vi "Array of VData to VArray__ogtk.vi"(7 "Array Name":string, 8 "error in (no error)":errorcluster, 9 "Element Type (when empty)":variant, 10 "1D Array of VData":variant[](array[variant])) -> (0 "error out":errorcluster, 2 "VArray":variant)   [LabVIEW 2023, in "openg_variant.lvlib"]
doc: "Converts a 1D Array of variants (of identical element datatypes) to an array of data wrapped in a Variant."
uses:
  openg_variant.lvlib
  error/error.llb/openg_error.lvlib
panel:
  # "[OpenG VI Tags] ***Do Not Remove***"
  # "Array of VData to VArray.vi\n\nConverts a 1D Array of variants (of identical element datatypes) to an array of \n\nPlease visit http://www.OpenG.org to learn about the\nOpen Source LabVIEW software movement.\n\nNOTICE -- YOU MUST LEAVE THIS NOTICE IN PLACE.  PER THE TERMS OF THE LICENSE BELOW, YOU MAY SUBLICENSE THIS SOFTWARE \nIN ANY WAY THAT DOES NOT CONFLICT WITH THIS LICENSE.\n\n### BSD License (http://www.opensource.org/licenses/bsd-license.php) Begin ###\n \nCopyright (c) 2002, Jean-Pierre Drolet <drolet_jp@hotmail.com>\nCopyright (c) 2002-2006, Jim Kring <jim@jimkring.com>\n\nAll rights reserved.\n\nRedistribution and use in source and binary forms, with or without modification, are permitted provided that the following conditions are met:\n\n    * Redistributions of source code must retain the above copyright notice, this list of conditions and the following disclaimer.\n    * Redistributions in binary form must reproduce the above copyright notice, this list of conditions and the following disclaimer in the \n       documentation and/or other materials provided with the distribution.\n    * Neither the name of SciWare, James Kring, Inc., nor the names of its contributors may be used to endorse or promote products derived \n       from this software without specific prior written permission.\n\nTHIS SOFTWARE IS PROVIDED BY THE COPYRIGHT HOLDERS AND CONTRIBUTORS \"AS IS\" AND ANY EXPRESS OR IMPLIED WARRANTIES, \nINCLUDING, BUT NOT LIMITED TO, THE IMPLIED WARRANTIES OF MERCHANTABILITY AND FITNESS FOR A PARTICULAR PURPOSE ARE \nDISCLAIMED. IN NO EVENT SHALL THE COPYRIGHT OWNER OR CONTRIBUTORS BE LIABLE FOR ANY DIRECT, INDIRECT, INCIDENTAL,\n SPECIAL, EXEMPLARY, OR CONSEQUENTIAL DAMAGES (INCLUDING, BUT NOT LIMITED TO, PROCUREMENT OF SUBSTITUTE GOODS OR \nSERVICES; LOSS OF USE, DATA, OR PROFITS; OR BUSINESS INTERRUPTION) HOWEVER CAUSED AND ON ANY THEORY OF LIABILITY, \nWHETHER IN CONTRACT, STRICT LIABILITY, OR TORT (INCLUDING NEGLIGENCE OR OTHERWISE) ARISING IN ANY WAY OUT OF THE USE \nOF THIS SOFTWARE, EVEN IF ADVISED OF THE POSSIBILITY OF SUCH DAMAGE.\n\n### BSD License End ###"
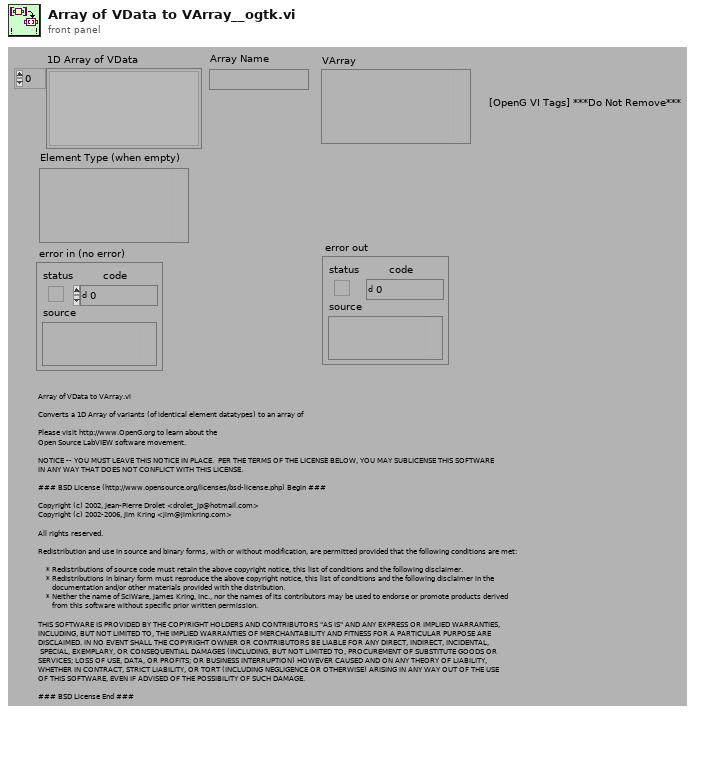
[diagram p1: front panel]
types:
  T1 = typedef "openg_variant.lvlib/Type Descriptor Enumeration__ogtk.ctl" = enum8{"<Null>", "I8", "I16", "I32", "I64", "U8", "U16", "U32", "U64", "SGL", "DBL", "EXT", "CSG", "CDB", "CXT", "0x0F", "0x10", "0x11", "0x12", "0x13", "0x14", "Enum U8", "Enum U16", "Enum U32", "Enum U64", "SGL PQ", "DBL PQ", "EXT PQ", "CSG PQ", "CDB PQ", "CXT PQ", "0x1F", "0x20", "Boolean", "0x22", "0x23", "0x24", "0x25", "0x26", "0x27", "0x28", "0x29", "0x2A", "0x2B", "0x2C", "0x2D", "0x2E", "0x2F", "String", "0x31", "Path", "Pict", "0x34", "0x35", "0x36", "DAQ", "0x38", "0x39", "0x3A", "0x3B", "0x3C", "0x3D", "0x3E", "0x3F", "Array", "0x41", "0x42", "0x43", "0x44", "0x45", "0x46", "0x47", "0x48", "0x49", "0x4A", "0x4B", "0x4C", "0x4D", "0x4E", "0x4F", "Cluster", "0x51", "0x52", "Variant", "Waveform", "0x55", "0x56", "0x57", "0x58", "0x59", "0x5A", "0x5B", "0x5C", "0x5D", "0x5E", "Fixed Point", "0x60", "0x61", "0x62", "0x63", "0x64", "0x65", "0x66", "0x67", "0x68", "0x69", "0x6A", "0x6B", "0x6C", "0x6D", "0x6E", "0x6F", "Refnum", "0x71", "0x72", "Set Collection", "Map Collection"}
  T2 = typedef "openg_variant.lvlib/Type Descriptor__ogtk.ctl" = i16[]
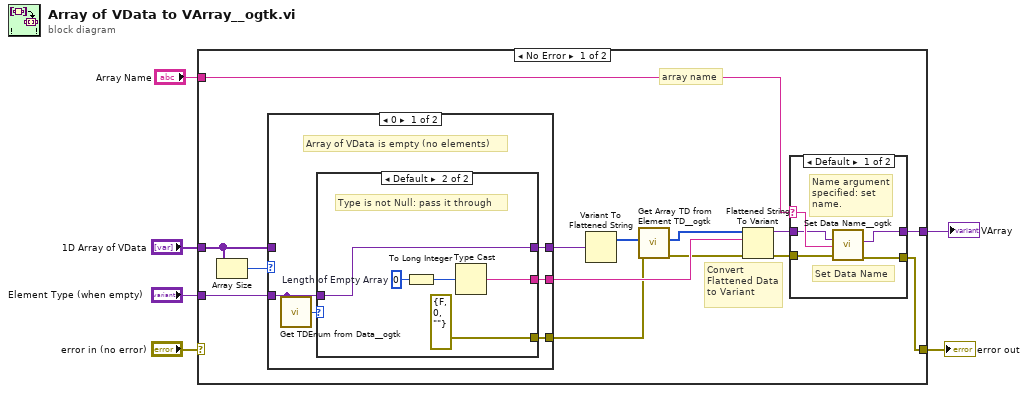
[diagram p0: block diagram]
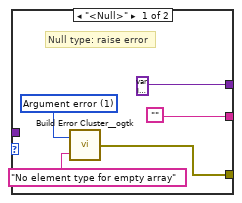
[diagram p2: hidden frame]
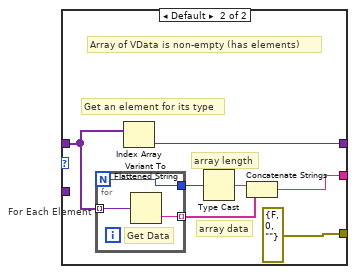
[diagram p3: hidden frame]
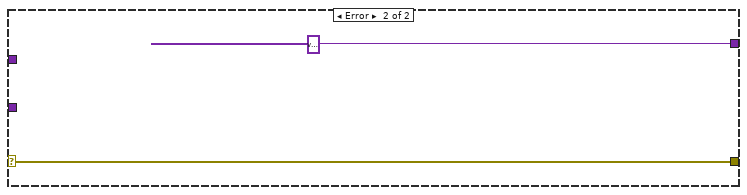
[diagram p5: hidden frame]
diagram:
  n1 = case shown="No Error" "error in (no error)" {
    selector: "error in (no error)" -> [_ w54]
    tunnel: [w14 variant ("VArray")] -> w3
    tunnel: [w12 w54] -> w2
    tunnel: "1D Array of VData" -> [w20 _]
    tunnel: "Element Type (when empty)" -> [w18 _]
    tunnel: "Array Name" -> [w11 _]
    frame No Error {
      # "array name"
      # "Convert Flattened Data to Variant"
      n2 = Array Size(array=w20) -> (size(s)=w19:i32)
      n3 = case shown="0" w19 {
        tunnel: [w23 w42] -> w17
        tunnel: [w24 errorcluster {"status"=FALSE, "code"=0, "source"=""} ("error out")] -> w8
        tunnel: w20 -> [_ w40]
        tunnel: w18 -> [w22 _]
        tunnel: [w21 w36] -> w16
        frame 0 {
          # "Array of VData is empty (no elements)"
          n4 = call "Get TDEnum from Data__ogtk.vi"("Data"=w22) -> ("Type Descriptor Enumeration"=w25:T1)  [unwired: 4 in]
          n5 = case shown="Default" w25 {
            tunnel: [w30 errorcluster {"status"=FALSE, "code"=0, "source"=""} ("error out")] -> w24
            tunnel: [variant ("Element Type (when empty)") w35] -> w23
            tunnel: w22 -> [_ w35]
            tunnel: ["" w32] -> w21
            frame "<Null>" {
              w29 = 1 items=["No error", "Argument error", "Memory is full", "Out of zone", "End of file", "File already open", "Generic file I/O error", "File not found", "File permission error", "Disk is full", "Duplicate path", "Too many files open", "System feature not enabled", "Resource file not found", "Cannot add resource", "Resource not found", "Image not found", "Image memory error", "Pen does not exist", "Config type invalid", "Config token not found", "Config parse error", "Config memory error", "Bad external code format", "Bad external code offset", "External code not present", "Null window", "Destroy window error", "Null menu", "Print aborted", "Bad print record", "Print driver error", "Windows error during printing", "Memory error during printing", "Print dialog error", "Generic print error", "Invalid device refnum", "Device not found", "Device parameter error", "Device unit error", "Cannot open device", "Device call aborted", "Generic error", "Cancelled by user", "Object ID too low", "Object ID too high", "Object not in heap", "Unknown heap", "Unknown object (invalid DefProc)", "Unknown object (DefProc not in table)", "Message out of range", "Invalid (null) method", "Unknown message", "Manager call not supported", "Bad address", "Network operation in progress", "Network operation timed out", "Connection is busy", "Network attribute not supported", "Network error", "Address in use", "System out of memory", "Connection aborted", "Connection refused", "Not connected", "Already connected", "Connection closed", "Initialization error (interapplication manager)", "Bad occurrence", "Wait on unbound occurrence handler", "Occurrence queue overflow", "Datalog type conflict", "Unused", "Unrecognized type (interapplication manager)", "Memory corrupt", "Failed to make temporary DLL", "Old CIN version", "Drag socket not found", "Failed to load drop-object", "Failed to register OLE object", "Failed to release OLE object", "Format specifier type mismatch", "Unknown format specifier", "Too few format specifiers", "Too many format specifiers", "Scan failed", "Newer CIN version", "Error converting to variant", "Runtime menu error", "Password tampered", "Variant attribute not found", "Incompatible variant data type", "Event data is not available", "Event Store is not present", "Occurrence is not found", "Event Queue is not created", "Event info is not available", "Refnum passed is NULL", "Error retrieving Class GUID", "Error retrieving CoClass GUID", "Error retrieving TypeLib GUID.", "Bad built application magic bytes.", "Specific driver is different from the specific driver associated with the Logical Name.", "There is no session opened to the class driver.", "Max Error", "MAX - Error with config objects", "MAX - Error loading configuration", "MAX - Group not supported"]
              # "Null type: raise error"
              n6 = call "Build Error Cluster__ogtk.vi"("String to Prepend to source (\"\")"="No element type for empty array" ("String to Prepend to source (\"\")"), "code"=w29) -> ("error out"=w30:errorcluster)
            }
            frame Default {
              w33 = 0  # Length of Empty Array
              # "Type is not Null: pass it through"
              n7 = To Long Integer(number=w33) -> (32bit integer=w31:i32)
              n8 = Type Cast(x=w31) -> (*(type *) &x=w32:string)  [unwired: 1 in]
            }
          }
        }
        frame Default {
          # "Get an element for its type"
          # "array length"
          # "array data"
          # "Array of VData is non-empty (has elements)"
          n9 = for "For Each Element" {
            N -> [w43]
            tunnel: w40 -> [w45] mode=indexing
            tunnel: [w44] -> w39 mode=indexing
            tunnel: [w43] -> w37
            # "Get Data"
            n10 = Variant To Flattened String(Variant=w45) -> (data string=w44:string)  [unwired: 1 out]
          }
          n11 = Index Array(array=w40) -> (element=w42:variant)  [unwired: 1 in]
          n12 = Type Cast(x=w37) -> (*(type *) &x=w38:string)  [unwired: 1 in]
          n13 = Concatenate Strings(w38, w39) -> (w36:string)
        }
      }
      n14 = Variant To Flattened String(Variant=w17) -> (1:w10:i16[])  [unwired: 1 out]
      n15 = call "Get Array TD from Element TD__ogtk.vi"("error in (no error)"=w8, "Element Type Descriptor"=w10) -> ("error out"=w7:errorcluster, "Array Type Descriptor"=w9:T2)  [unwired: 8 in]
      n16 = Flattened String To Variant(4:w7, 6:w16, 7:w9) -> (0:w13:errorcluster, 3:w15:variant)
      n17 = case shown="Default" w11 {
        selector: w11 -> [w48 _]
        tunnel: [w46 w52] -> w14
        tunnel: w15 -> [w47 w52]
        tunnel: [w49 w51] -> w12
        tunnel: w13 -> [w50 w51]
        frame Default {
          # "Name argument specified: set name."
          # "Set Data Name"
          n18 = call "Set Data Name__ogtk.vi"("error in (no error)"=w50, "Data Name"=w48, "Data"=w47) -> ("error out"=w49:errorcluster, "Renamed Data"=w46:variant)  [unwired: 7 in]
        }
        frame "" {
          # "Name argument is empty: don't set name."
        }
      }
    }
    frame Error {
    }
  }
  "VArray" <- w3
  "error out" <- w2
